vi "Format Potting Points.vi"(8 "error in":errorcluster, 9 "WorkTable":refnum<class "WorkTable Class.lvclass">, 10 "Array":T1[](array[typedef]), 11 "Console Log in":refnum<class "Console Log.lvclass">) -> (0 "error out":errorcluster, 2 "Formatted Potting Points":string, 3 "Console Log out":refnum<class "Console Log.lvclass">)   [LabVIEW 2011, in "Console Log.lvclass"]
uses:
  Console Log.lvclass
  Shared Components/SyringeTool Class/Type Definitions/Module Potting Data.ctl
  Shared Components/Vec3d Class/Vec3d Class.lvclass
  Shared Components/Utils/Type Definitions/3d Line.ctl
  Shared Components/Utils/Type Definitions/3d Point.ctl
  Shared Components/WorkTable Class/WorkTable Class.lvclass
  Shared Components/Config Manager Class/Type Definitions/Part Type.ctl
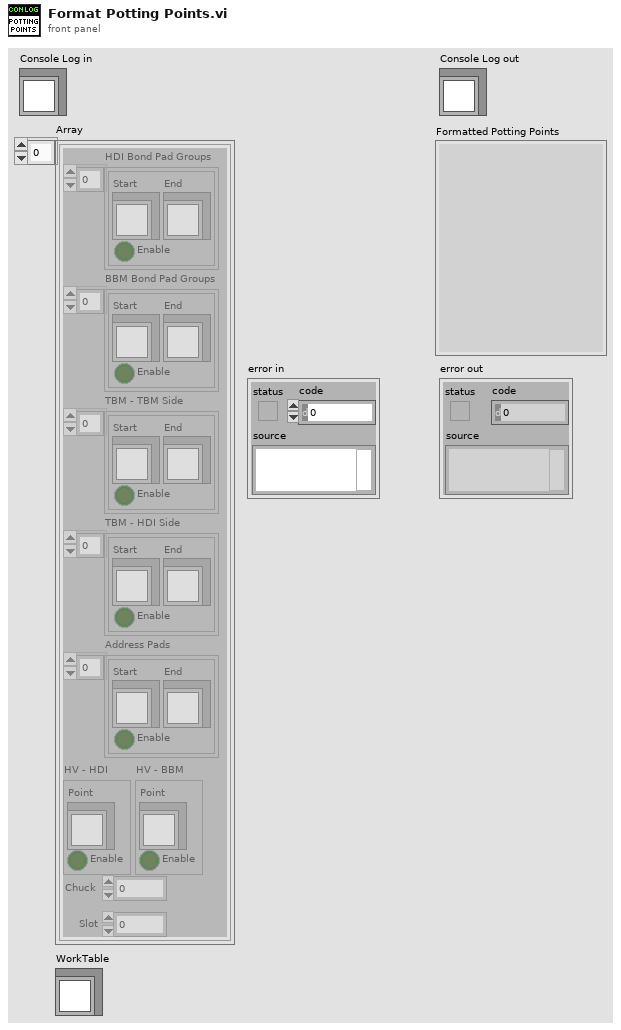
[diagram p1: front panel]
types:
  T1 = typedef "Module Potting Data.ctl" = cluster{"HDI Bond Pad Groups":T2[], "BBM Bond Pad Groups":T2[], "TBM - TBM Side":T2[], "TBM - HDI Side":T2[], "Address Pads":T2[], "Chuck":i32, "Slot":i32, "HV - HDI":T3, "HV - BBM":T3}
  T2 = typedef "3d Line.ctl" = cluster{"Start":refnum<class "Vec3d Class.lvclass">, "End":refnum<class "Vec3d Class.lvclass">, "Enable":bool}
  T3 = typedef "3d Point.ctl" = cluster{"Point":refnum<class "Vec3d Class.lvclass">, "Enable":bool}
  T4 = typedef "Part Type.ctl" = enum16{"BBM", "HDI", "BARE HDI", "GLUERESERVOIR", "STAMP_1", "STAMP_2", "STAMP_3", "STAMP_4", "STAMP_5", "WEIGHT_1", "WEIGHT_2", "WEIGHT_3", "WEIGHT_4", "WEIGHT_5", "WEIGHT_6", "WEIGHT_7", "WEIGHT_8", "PICKER_TOOL", "GRABER_TOOL"}
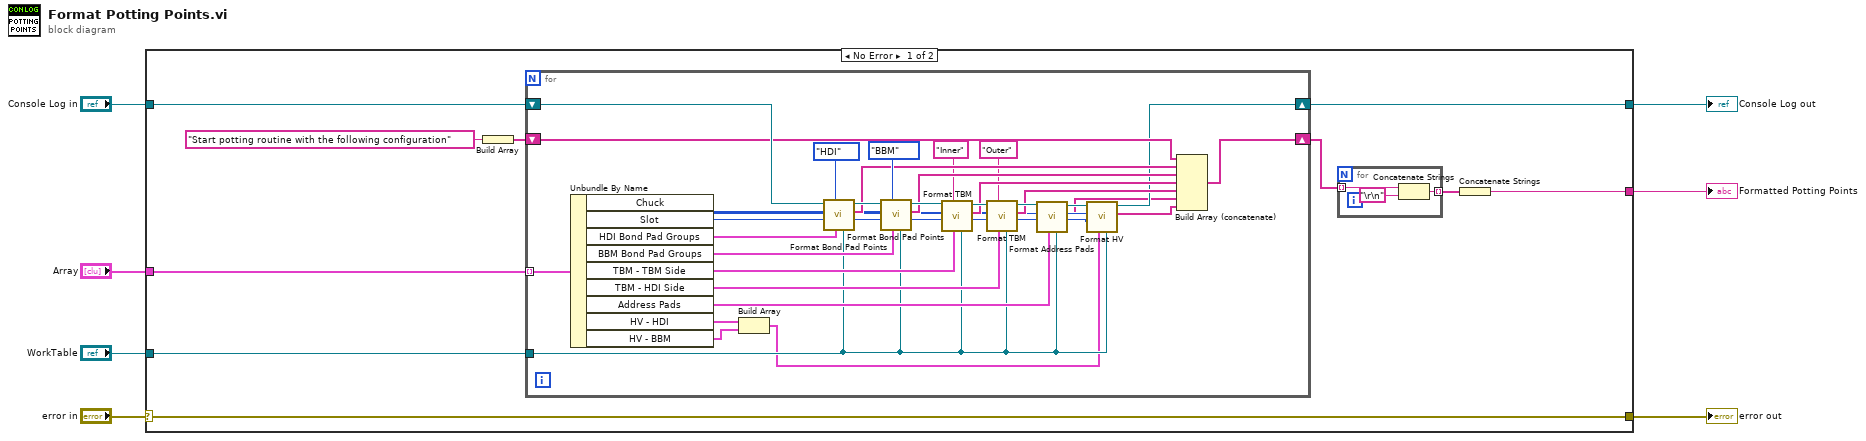
[diagram p0: block diagram]
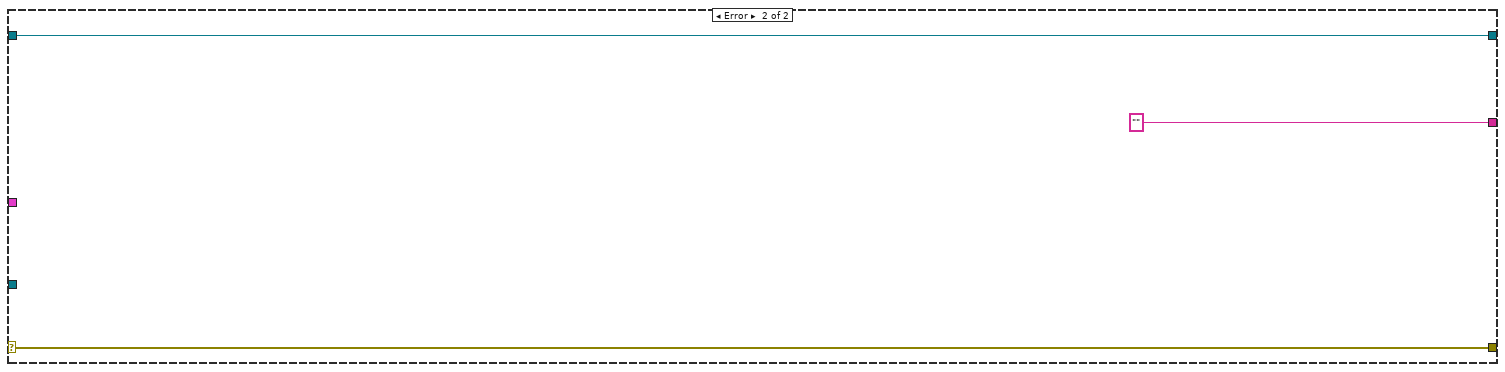
[diagram p2: hidden frame]
diagram:
  n1 = case shown="No Error" "error in" {
    selector: "error in" -> [w11 w54]
    tunnel: [w11 w54] -> w6
    tunnel: [w9 w53] -> w4
    tunnel: "Console Log in" -> [w12 w53]
    tunnel: "Array" -> [w16 _]
    tunnel: [w10 ""] -> w2
    tunnel: "WorkTable" -> [w8 _]
    frame No Error {
      n2 = Build Array("Start potting routine with the following configuration") -> (w15:string[])
      n3 = for {
        tunnel: w16 -> [w51] mode=indexing
        shift-right: [w34] -> w14
        shift-left: w15 -> [w33]
        shift-right: [w27] -> w9
        shift-left: w12 -> [w48]
        tunnel: w8 -> [w22]
        n4 = Unbundle By Name(w51) -> ("Chuck"=w26:i32, "Slot"=w25:i32, "HDI Bond Pad Groups"=w50:T2[], "BBM Bond Pad Groups"=w45:T2[], "TBM - TBM Side"=w43:T2[], "TBM - HDI Side"=w41:T2[], "Address Pads"=w40:T2[], "HV - HDI"=w30:T3, "HV - BBM"=w29:T3)
        n5 = Build Array(w30, w29) -> (w21:T3[])
        n6 = call "Format Bond Pad Points.vi"("WorkTable"=w22, "Bond Pad Groups"=w50, "Part Type"=Part_Type."HDI", "Slot"=w25, "Chuck"=w26, "Console Log in"=w48) -> ("Formatted Bond Pads"=w38:string[], "Console Log out"=w47:refnum<class "Console Log.lvclass">)  [unwired: 3 in, 1 out]
        n7 = call "Format Bond Pad Points.vi"("WorkTable"=w22, "Bond Pad Groups"=w45, "Part Type"=Part_Type."BBM", "Slot"=w25, "Chuck"=w26, "Console Log in"=w47) -> ("Formatted Bond Pads"=w37:string[], "Console Log out"=w44:refnum<class "Console Log.lvclass">)  [unwired: 3 in, 1 out]
        n8 = call "Format TBM.vi"("WorkTable"=w22, "Bond Pad Groups"=w43, "Inner/Outer"="Inner", "Slot"=w25, "Chuck"=w26, "Console Log in"=w44) -> ("Formatted TBM"=w36:string[], "Console Log out"=w42:refnum<class "Console Log.lvclass">)  [unwired: 3 in, 1 out]
        n9 = call "Format TBM.vi"("WorkTable"=w22, "Bond Pad Groups"=w41, "Inner/Outer"="Outer", "Slot"=w25, "Chuck"=w26, "Console Log in"=w42) -> ("Formatted TBM"=w35:string[], "Console Log out"=w39:refnum<class "Console Log.lvclass">)  [unwired: 3 in, 1 out]
        n10 = call "Format Address Pads.vi"("WorkTable"=w22, "Sides"=w40, "Slot"=w25, "Chuck"=w26, "Console Log in"=w39) -> ("Formatted Address Pads"=w24:string[], "Console Log out"=w28:refnum<class "Console Log.lvclass">)  [unwired: 4 in, 1 out]
        n11 = call "Format HV.vi"("WorkTable"=w22, "HV Points"=w21, "Slot"=w25, "Chuck"=w26, "Console Log in"=w28) -> ("Formatted Address Pads"=w23:string[], "Console Log out"=w27:refnum<class "Console Log.lvclass">)  [unwired: 4 in, 1 out]
        n12 = Build Array (concatenate)(w33, w38, w37, w36, w35, w24, w23) -> (w34:string[])
      }
      n13 = for {
        tunnel: w14 -> [w19] mode=indexing
        tunnel: [w20] -> w13 mode=indexing
        n14 = Concatenate Strings(w19, "\r\n") -> (w20:string)
      }
      n15 = Concatenate Strings(w13) -> (w10:string)
    }
    frame Error {
    }
  }
  "error out" <- w6
  "Console Log out" <- w4
  "Formatted Potting Points" <- w2
